vi "conversionsGraph (SubVI).vi"(4 "K0":dbl, 5 "Array":dbl[](array[numeric]), 6 "Offset":dbl, 7 "Array in":T2(array[cluster]), 8 "Numeric":dbl, 9 "Gain":dbl, 10 "K1":dbl, 11 "RH/T Sensor VSS (V)":dbl) -> (3 "Cluster":T1)   [LabVIEW 2014]
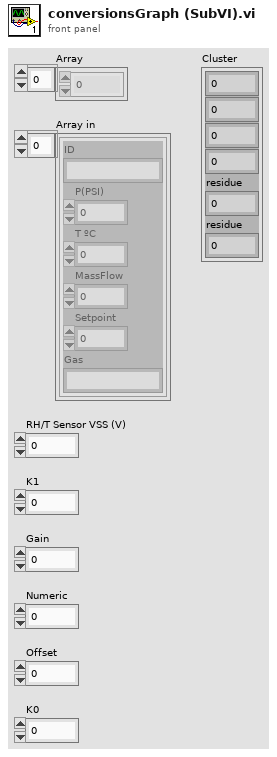
[diagram p1: front panel]
types:
  T1 = cluster{dbl, dbl, dbl, dbl, "residue":dbl, "residue":dbl}
  T2 = cluster{"ID":string, "P(PSI)":dbl, "T ºC":dbl, "MassFlow":dbl, "Setpoint":dbl, "Gas":string}[]
  T3 = cluster{"Numeric":dbl, dbl, dbl, dbl, "residue":dbl, "residue":dbl}
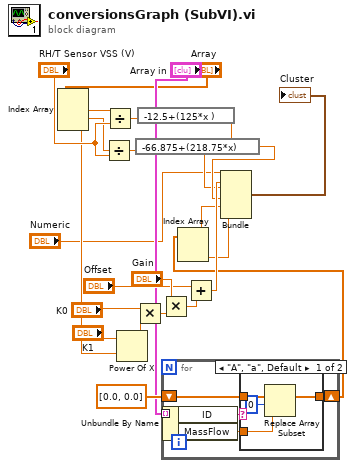
[diagram p0: block diagram]
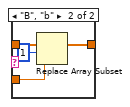
[diagram p2: hidden frame]
diagram:
  n1 = Index Array(array="Array") -> (element #1=w9:dbl, element #2=w10:dbl, element #3=w22:dbl)  [unwired: 3 in]
  n2 = Divide(x=w10, y="RH/T Sensor VSS (V)") -> (x/y=w13:dbl)
  n3 = Divide(x=w9, y="RH/T Sensor VSS (V)") -> (x/y=w11:dbl)
  n4 = Power Of X(1:w22, 2:"K1") -> (0:w21:dbl)
  n5 = Multiply(x="K0", y=w21) -> (x*y=w20:dbl)
  n6 = expression code="-66.875+(218.75*x)"(w13) -> (w14:dbl)
  n7 = expression code="-12.5+(125*x )"(w11) -> (w12:dbl)
  n8 = Multiply(x="Gain", y=w20) -> (x*y=w19:dbl)
  n9 = for {
    tunnel: "Array in" -> [w29] mode=indexing
    shift-right: [w26] -> w6
    shift-left: dbl[] [0.0, 0.0] -> [w27]
    n10 = Unbundle By Name(w29) -> ("ID"=w28:string, "MassFlow"=w25:dbl)
    n11 = case shown="\"A\", \"a\", Default" w28 {
      tunnel: [w33 w37] -> w26
      tunnel: w27 -> [w32 w36]
      tunnel: w25 -> [w31 w35]
      frame "A", "a", Default {
        n12 = Replace Array Subset(array=w32, new element=w31, index=0) -> (w33:dbl[])
      }
      frame "B", "b" {
        n13 = Replace Array Subset(array=w36, new element=w35, index=1) -> (w37:dbl[])
      }
    }
  }
  n14 = Index Array(array=w6) -> (element #1=w7:dbl, element #2=w8:dbl)  [unwired: 2 in]
  n15 = Add(x="Offset", y=w19) -> (x+y=w23:dbl)
  n16 = Bundle("Numeric"="Numeric", w23, w12, w14, "residue"=w7, "residue"=w8) -> (→"Cluster":T3)  [unwired: 1 in]
